vi "Dig Grave Test.vi"   [LabVIEW 2017, in "Tests.lvlib"]
uses:
  Tests.lvlib
  src/Eulogy/Eulogy.lvlib
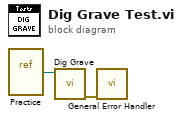
[diagram p0: block diagram]
diagram:
  n1 = vi-ref "Practice.vi"() -> (w2:refnum<vi>)
  n2 = call "Dig Grave.vi"("VI In"=w2) -> ("Error Out"=w1:errorcluster)  [unwired: 9 in, 1 out]
  n3 = call <vilib>:"General Error Handler.vi"("error in (no error)"=w1) -> ()  [unwired: 10 in, 5 out]
